vi "ConfigurationFileWrite.vi"() -> ()   [LabVIEW 2016]
uses:
  controls/Enum.ctl
  <vilib>/Utility/config.llb/Write Key (String).vi
  <vilib>/Utility/config.llb/Write Key (Double).vi
  <vilib>/Utility/config.llb/Write Key (Boolean).vi
  <vilib>/Utility/config.llb/Write Key (U32).vi
  <vilib>/Utility/config.llb/Write Key (I32).vi
  <vilib>/Utility/config.llb/NI_LVConfig.lvlib
  <vilib>/Utility/config.llb/Write Key (Path).vi
panel:
  in  "default name":path=path "Configuration File3.ini"
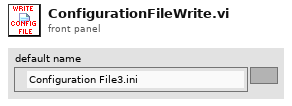
[diagram p1: front panel]
types:
  T1 = typedef "NI_LVConfig.lvlib/Config Data RefNum.ctl" = refnum<k1>
  T2 = typedef "Enum.ctl" = enum16{"Init", "Read", "Write"}
  T3 = enum16{"fractional", "engineering", "exponential"}
  T4 = enum16{"Vert. Deflection", "Horiz. Deflection", "Amplitude", "..."}
  T5 = enum32{"No Selection", "FullScale", "Standard Deviation"}
  T6 = cluster{i32, "Direction":enum16{"Forward", "Backward"}, "Processing":enum16{"None", "Offset", "Line", "Polynom"}, "Color":enum16{"Blue", "Gray", "Gold", "Green", "Red", "Asylum", "Adrian", "Nanoscope", "NanoscopeIII"}}
  T7 = enum32{"Invalid", "Standard", "Closed", "Hidden", "Minimized", "Maximized"}
  T8 = typedef "LVPositionTypeDef.ctl" = cluster{"Left":i32, "Top":i32}
  T9 = cluster{"calibName":string[], "calibParameters":cluster{"Sensitivity":cluster{"Sens X":dbl, "Sens Y":dbl, "Sens Z":dbl}, "Range":cluster{"Range X":dbl, "Range Y":dbl, "Range Z":dbl}, "HV gain":cluster{"HV gain X":dbl, "HV gain Y":dbl, "HV gain Z":dbl}}[], "calibIndex":i32}
  T10 = cluster{"Sensitivity":cluster{"Sens X":dbl, "Sens Y":dbl, "Sens Z":dbl}, "Range":cluster{"Range X":dbl, "Range Y":dbl, "Range Z":dbl}, "HV gain":cluster{"HV gain X":dbl, "HV gain Y":dbl, "HV gain Z":dbl}}[]
  T11 = cluster{"Sensitivity":cluster{"Sens X":dbl, "Sens Y":dbl, "Sens Z":dbl}, "Range":cluster{"Range X":dbl, "Range Y":dbl, "Range Z":dbl}, "HV gain":cluster{"HV gain X":dbl, "HV gain Y":dbl, "HV gain Z":dbl}}
  T12 = cluster{"Sens X":dbl, "Sens Y":dbl, "Sens Z":dbl}
  T13 = cluster{"Range X":dbl, "Range Y":dbl, "Range Z":dbl}
  T14 = cluster{"HV gain X":dbl, "HV gain Y":dbl, "HV gain Z":dbl}
  T15 = cluster{"ActiveController":dbl, "ControllerNames":string[], "ControllerParameters":cluster{"Controller Config":cluster{"Slope":bool, "Controller type":enum16{"Bipolar", "Absolute"}, "Controller name":string, "Control Signal name":string, "Signal":enum16{"Vert. Deflection", "Horiz. Deflection", "Amplitude", "..."}, "Unit":string}, "PID":cluster{"Setpoint":dbl, "P Gain":dbl, "I Gain":dbl}}[]}
  T16 = cluster{"Controller Config":cluster{"Slope":bool, "Controller type":enum16{"Bipolar", "Absolute"}, "Controller name":string, "Control Signal name":string, "Signal":enum16{"Vert. Deflection", "Horiz. Deflection", "Amplitude", "..."}, "Unit":string}, "PID":cluster{"Setpoint":dbl, "P Gain":dbl, "I Gain":dbl}}[]
  T17 = cluster{"Slope":bool, "Controller type":enum16{"Bipolar", "Absolute"}, "Controller name":string, "Control Signal name":string, "Signal":enum16{"Vert. Deflection", "Horiz. Deflection", "Amplitude", "..."}, "Unit":string}
  T18 = cluster{"Setpoint":dbl, "P Gain":dbl, "I Gain":dbl}
  T19 = typedef "ScanWaveform.ctl" = enum16{"Sine Wave", "Triangle Wave", "Rounded Wave"}
  T20 = cluster{"slowWavePts":u16, "fastWavePts":u16, "slowWaveType":T19, "fastWaveType":T19, "slowRoundPts":u16, "fastRoundPts":u16, "singleDirectionScan":bool}
  T21 = cluster{"Width":dbl, "Height":dbl, "X Offset":dbl, "Y Offset":dbl, "Angle":dbl, "Pixels/Line":u16, "Lines":u16, "Time/Line":dbl, "Scan Rate":dbl}
  T22 = enum16{"Blue", "Gray", "Gold", "Green", "Red", "Asylum", "Adrian", "Nanoscope", "NanoscopeIII"}
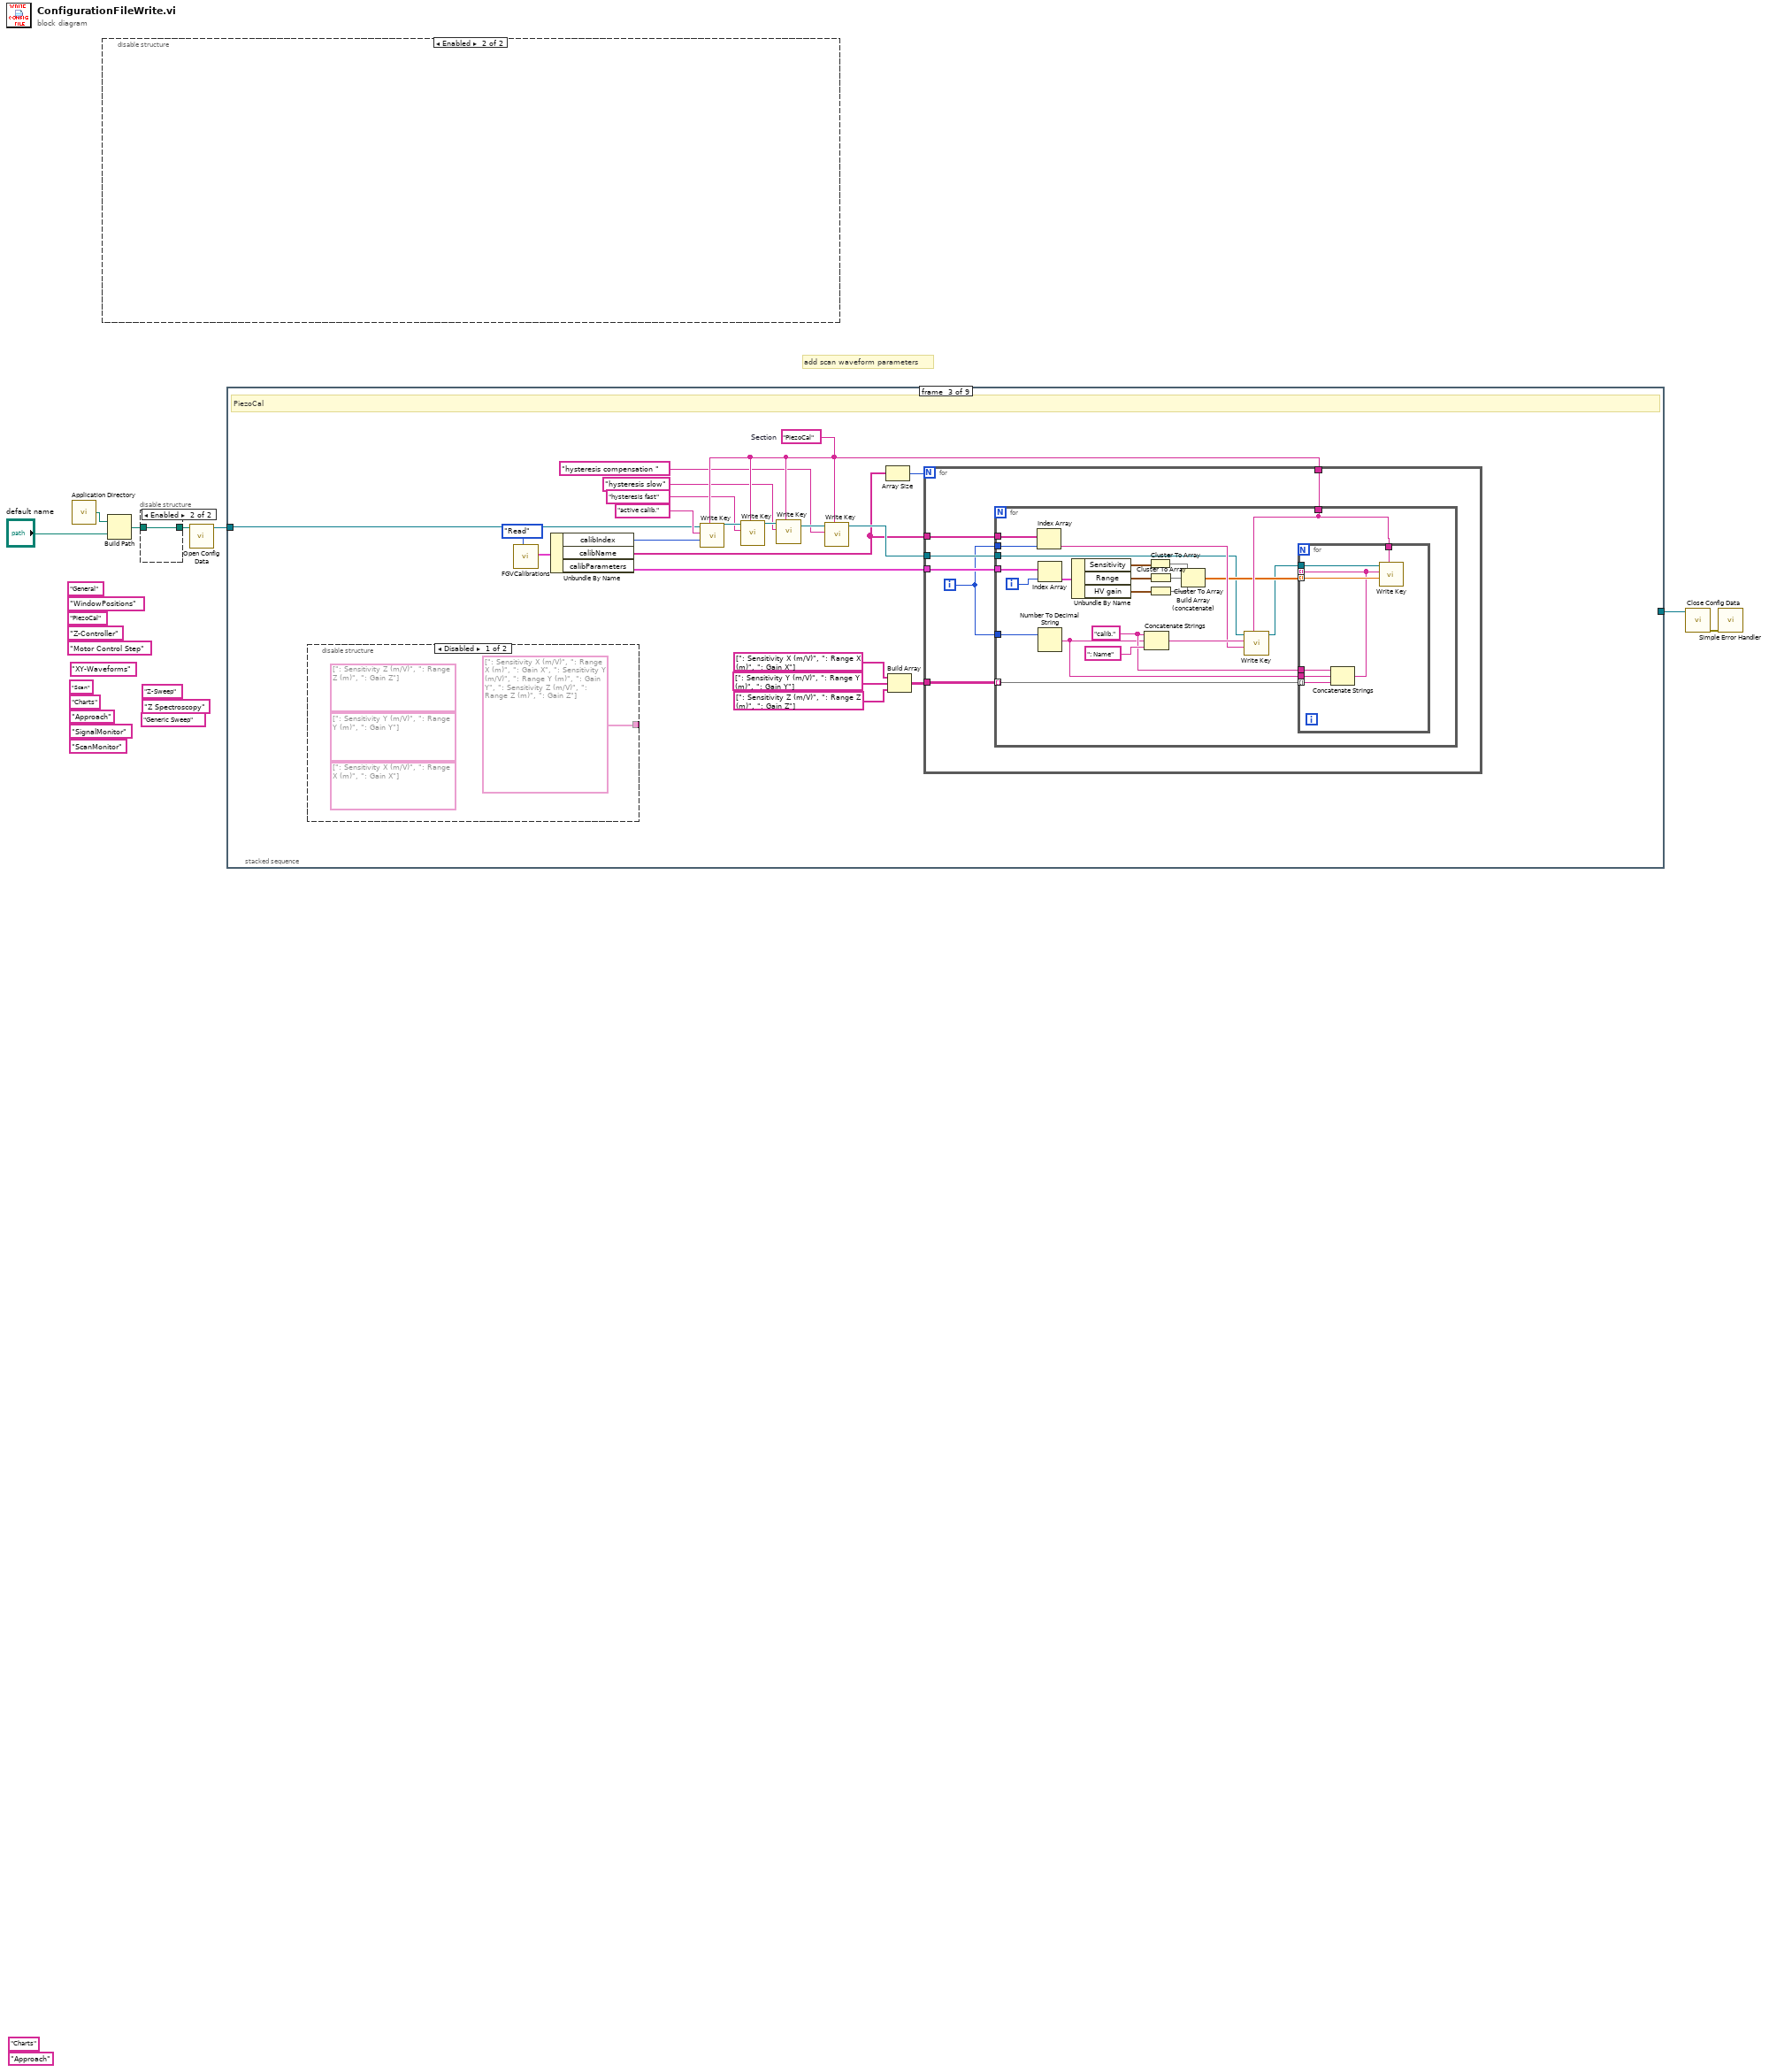
[diagram p0: block diagram]
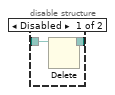
[diagram p2: hidden frame]
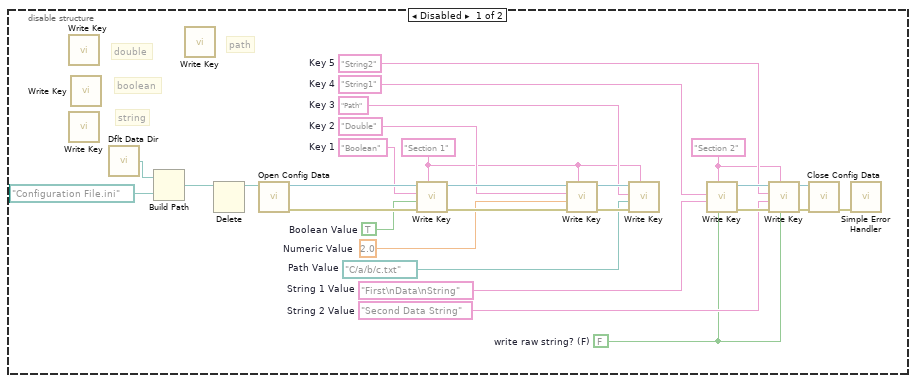
[diagram p3: hidden frame]
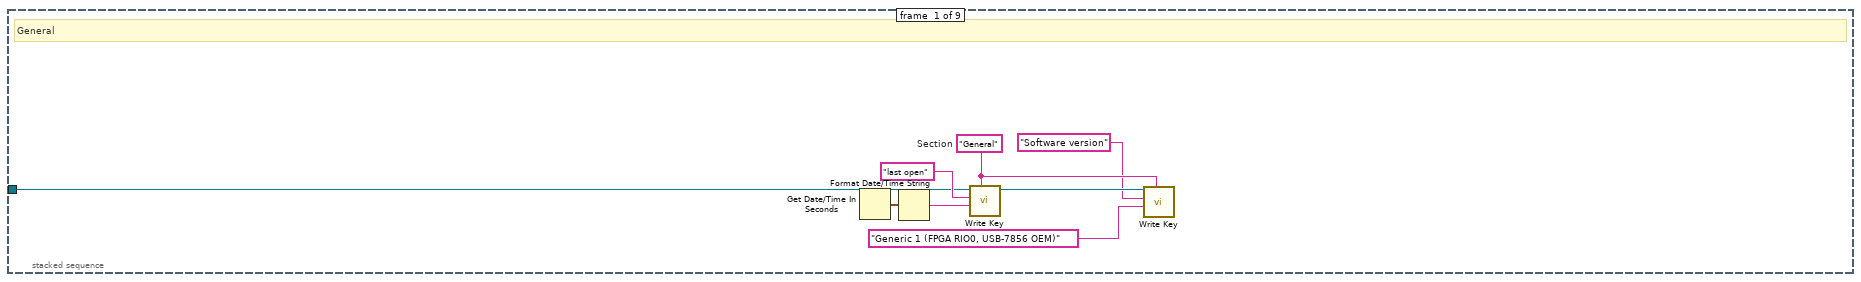
[diagram p4: hidden frame]
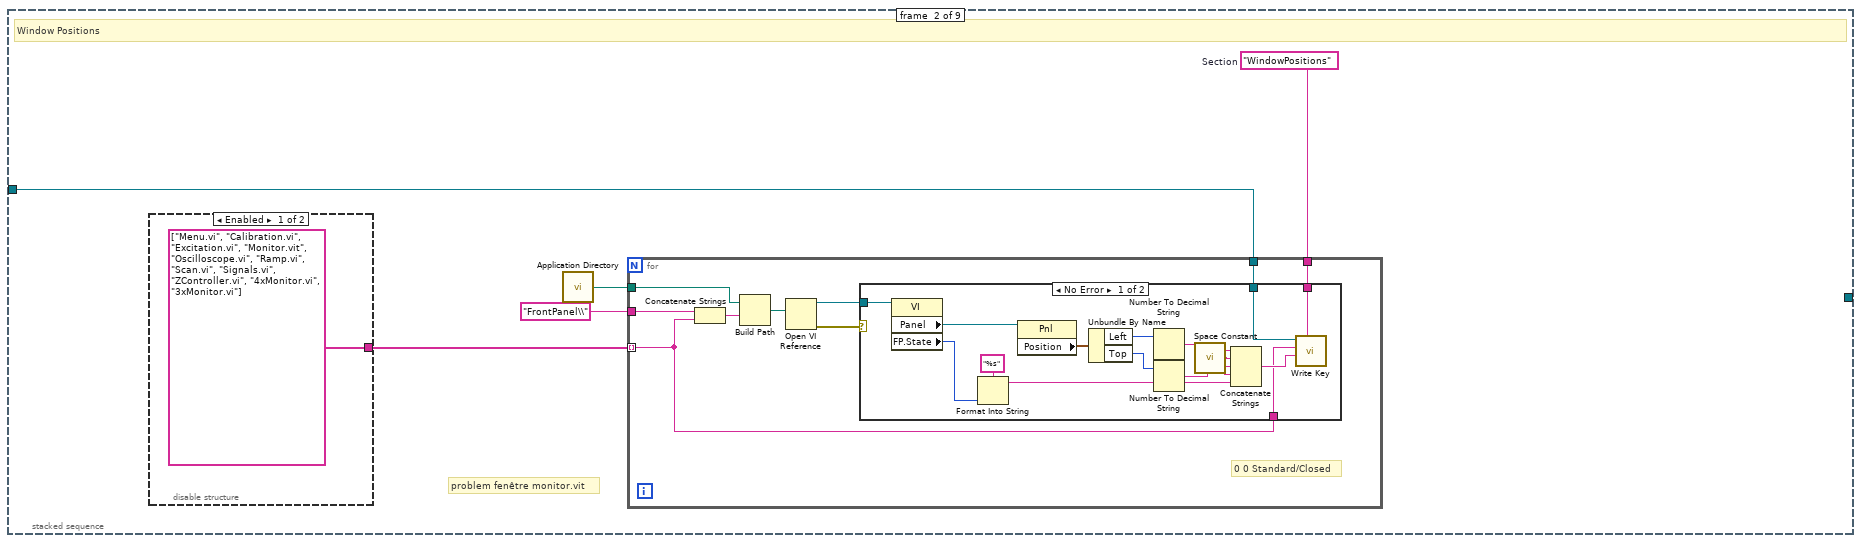
[diagram p5: hidden frame]
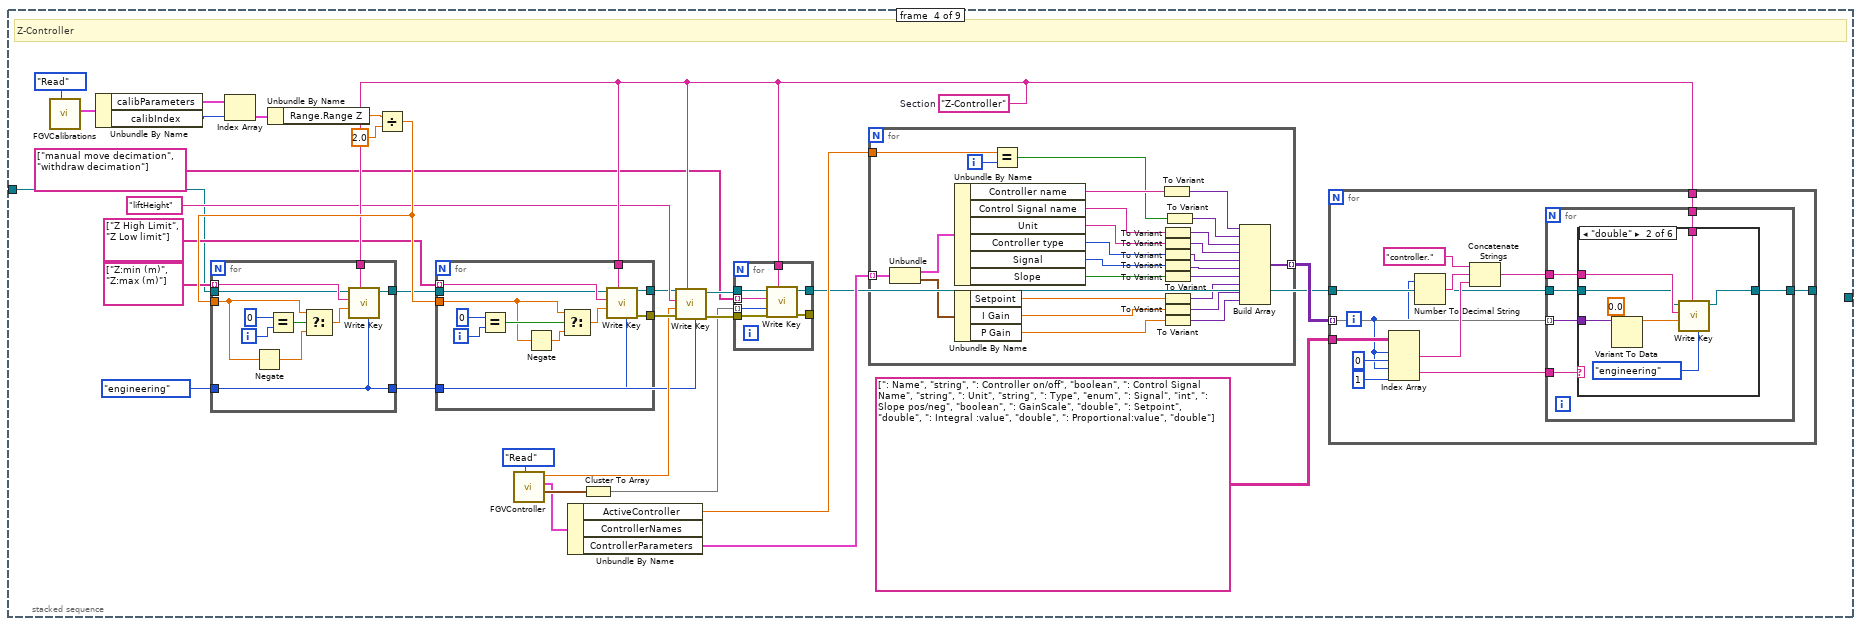
[diagram p9: hidden frame]
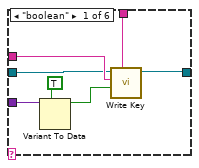
[diagram p10: hidden frame]
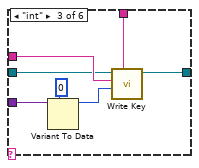
[diagram p11: hidden frame]
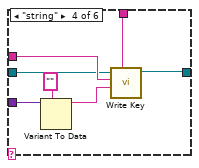
[diagram p12: hidden frame]
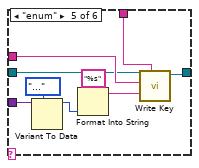
[diagram p13: hidden frame]
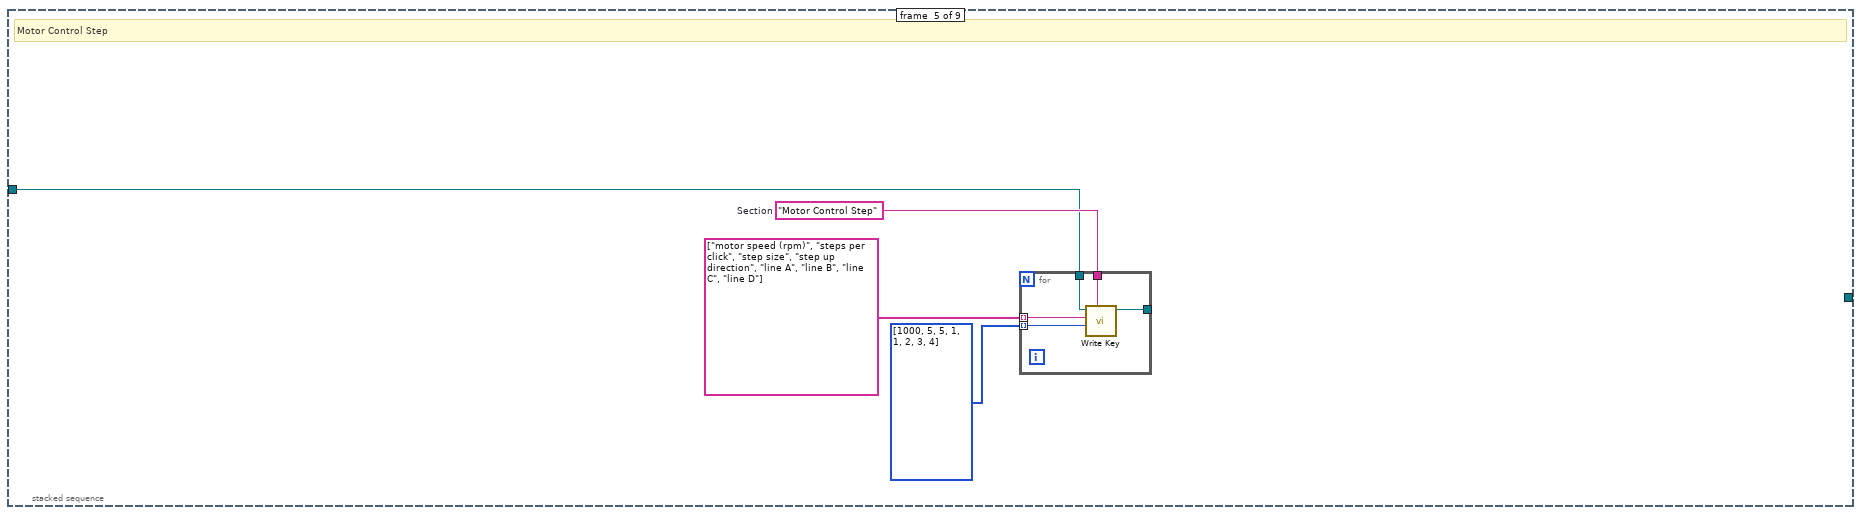
[diagram p15: hidden frame]
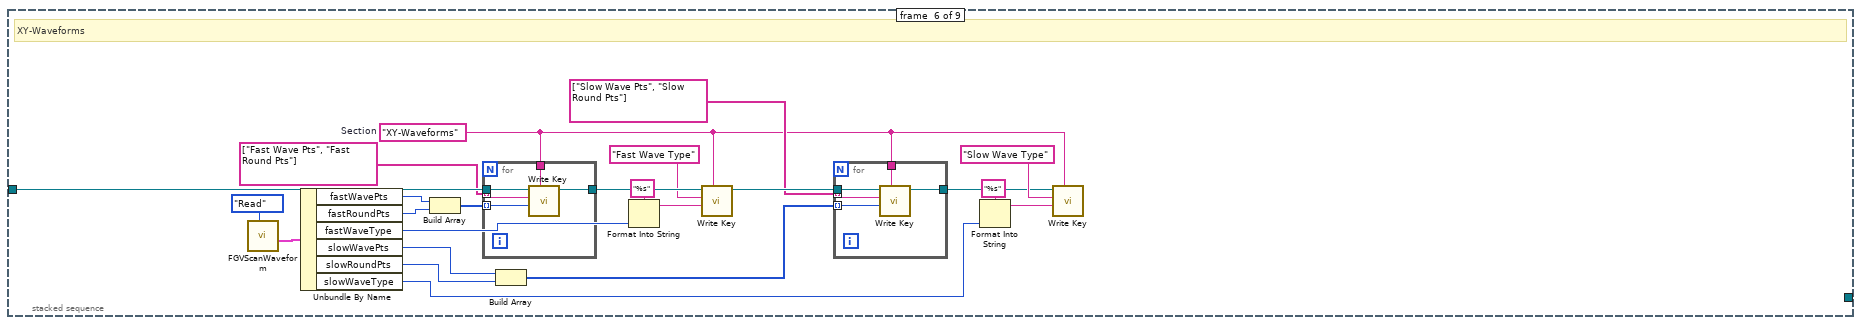
[diagram p16: hidden frame]
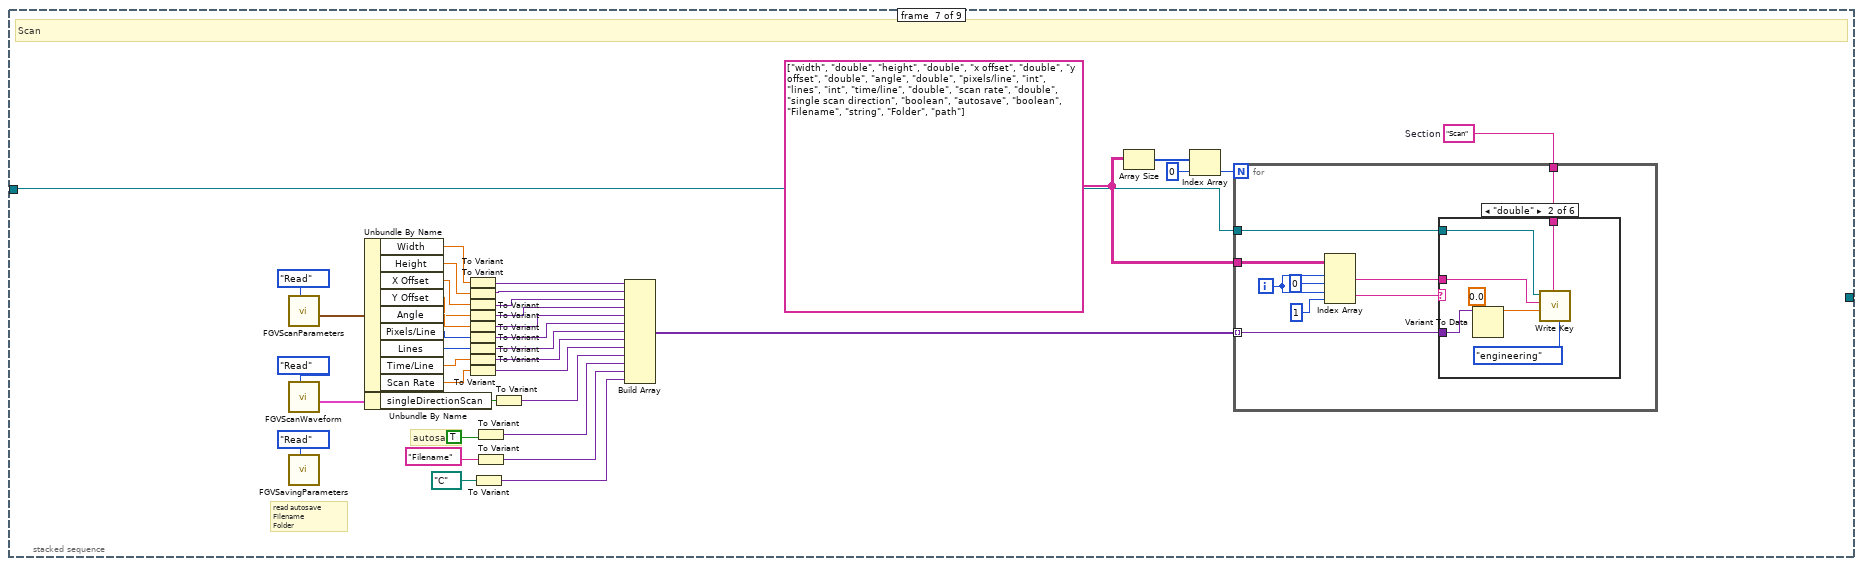
[diagram p17: hidden frame]
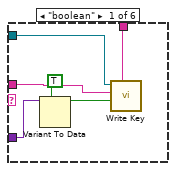
[diagram p18: hidden frame]
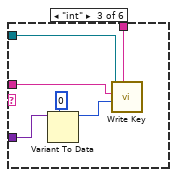
[diagram p19: hidden frame]
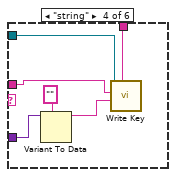
[diagram p20: hidden frame]
diagram:
  (unwired) "XY-Waveforms"
  (unwired) "Approach"
  (unwired) "Charts"
  (unwired) "Generic Sweep"
  (unwired) "ScanMonitor"
  (unwired) "Z Spectroscopy"
  (unwired) "Z-Sweep"
  (unwired) "SignalMonitor"
  (unwired) "Approach"
  (unwired) "Charts"
  (unwired) "Scan"
  (unwired) "Motor Control Step"
  (unwired) "Z-Controller"
  (unwired) "PiezoCal"
  (unwired) "WindowPositions"
  (unwired) "General"
  # "add scan waveform parameters"
  n1 = call <vilib>:"Application Directory.vi"() -> ("Application Directory"=w7:path)
  n2 = disable-structure shown="Enabled" {
    frame Disabled {
      w19 = "Second Data String"  # String 2 Value
      w20 = "First\nData\nString"  # String 1 Value
      w15 = path "C:/a/b/c.txt"  # Path Value
      w14 = 2.0  # Numeric Value
      w13 = TRUE  # Boolean Value
      w8 = FALSE  # write raw string? (F)
      w21 = "String2"  # Key 5
      w22 = "String1"  # Key 4
      w23 = "Path"  # Key 3
      w24 = "Double"  # Key 2
      w25 = "Boolean"  # Key 1
      w16 = "Section 2"
      w17 = "Section 1"
      # "string"
      # "path"
      # "boolean"
      # "double"
      n3 = call-poly <vilib>:"Write Key.vi"() -> ()  [unwired: 8 in, 4 out]
      n4 = call-poly <vilib>:"Write Key.vi"() -> ()  [unwired: 6 in, 6 out]
      n5 = call-poly <vilib>:"Write Key.vi"() -> ()  [unwired: 5 in, 7 out]
      n6 = call <vilib>:"Dflt Data Dir.vi"() -> ("App:Default Data Directory"=w11:path)
      n7 = Build Path(base path=w11, name or relative path=path "Configuration File.ini" ("default name")) -> (appended path=w9:path)
      n8 = call-poly <vilib>:"Write Key.vi"() -> ()  [unwired: 5 in, 7 out]
      n9 = Delete(path (use dialog)=w9) -> (deleted path=w10:path)  [unwired: 4 in, 2 out]
      n10 = call <vilib>:"Open Config Data.vi"("configuration file path"=w10) -> ("error out"=w30:errorcluster, "refnum"=w35:T1)  [unwired: 2 in, 7 out]
      n11 = call-poly <vilib>:"Write Key.vi"("section"=w17, "error in (no error)"=w30, "value"=w13, "key"=w25, "refnum"=w35) -> ("error out"=w29:errorcluster, "refnum out"=w34:T1)  [unwired: 5 out]
      n12 = call-poly <vilib>:"Write Key.vi"("section"=w17, "error in (no error)"=w29, "value"=w14, "key"=w24, "refnum"=w34) -> ("error out"=w28:errorcluster, "refnum out"=w33:T1)  [unwired: 3 in, 2 out]
      n13 = call-poly <vilib>:"Write Key.vi"("section"=w17, "error in (no error)"=w28, "value"=w15, "key"=w23, "refnum"=w33) -> ()  [unwired: 7 out]
      n14 = call-poly <vilib>:"Write Key.vi"("write raw string? (F)"=w8, "section"=w16, "value"=w20, "key"=w22) -> ("error out"=w27:errorcluster, "refnum out"=w32:T1)  [unwired: 2 in, 4 out]
      n15 = call-poly <vilib>:"Write Key.vi"("write raw string? (F)"=w8, "section"=w16, "error in (no error)"=w27, "value"=w19, "key"=w21, "refnum"=w32) -> ("error out"=w26:errorcluster, "refnum out"=w31:T1)  [unwired: 4 out]
      n16 = call <vilib>:"Close Config Data.vi"("error in (no error)"=w26, "refnum"=w31) -> ("error out"=w18:errorcluster)  [unwired: 1 in, 8 out]
      n17 = call <vilib>:"Simple Error Handler.vi"("error in (no error)"=w18) -> ()  [unwired: 1 in, 8 out]
    }
    frame Enabled {
    }
  }
  n18 = Build Path(base path=w7, name or relative path="default name") -> (appended path=w3:path)
  n19 = disable-structure shown="Enabled" {
    disable-tunnel: w3 -> [w37 w38]
    disable-tunnel: [w36 w38] -> w2
    frame Disabled {
      n20 = Delete(path (use dialog)=w37) -> (deleted path=w36:path)  [unwired: 4 in, 2 out]
    }
    frame Enabled {
    }
  }
  n21 = call <vilib>:"Open Config Data.vi"("configuration file path"=w2) -> ("refnum"=w6:T1)  [unwired: 2 in, 8 out]
  n22 = stacked-sequence {
    tunnel: w6 -> [w39 w48 w83 w136 w278 w309 w324 w404 w460]
    tunnel: [_ _ _ _ _ _ _ _ w459] -> w4
    frame #0 {
      w46 = "General"  # Section
      # "General"
      n23 = Get Date/Time In Seconds() -> (seconds since 1Jan1904=w44:timestamp)
      n24 = Format Date/Time String(seconds (now)=w44) -> (date/time string=w45:string)  [unwired: 2 in]
      n25 = call-poly <vilib>:"Write Key.vi"("section"=w46, "value"=w45, "key"="last open", "refnum"=w39) -> ("refnum out"=w43:T1)  [unwired: 2 in, 5 out]
      n26 = call-poly <vilib>:"Write Key.vi"("section"=w46, "value"="Generic 1 (FPGA RIO0, USB-7856 OEM)", "key"="Software version", "refnum"=w43) -> ()  [unwired: 2 in, 6 out]
    }
    frame #1 {
      w51 = "WindowPositions"  # Section
      # "problem fenêtre monitor.vit"
      # "Window Positions"
      n27 = disable-structure shown="Enabled" {
        disable-tunnel: [string[] ["Menu.vi", "Calibration.vi", "Excitation.vi", "Monitor.vit", "Oscilloscope.vi", "Ramp.vi", "Scan.vi", "Signals.vi", "ZController.vi", "4xMonitor.vi", "3xMonitor.vi"] _] -> w47
        frame Enabled {
        }
        frame Disabled {
        }
      }
      n28 = call <vilib>:"Application Directory.vi"() -> ("Application Directory"=w50:path)
      n29 = for {
        tunnel: "FrontPanel\\" ("string") -> [w61]
        tunnel: w50 -> [w58]
        tunnel: w47 -> [w57] mode=indexing
        tunnel: w51 -> [w56]
        tunnel: w48 -> [w54]
        # "0 0 Standard/Closed"
        n30 = Concatenate Strings(w61, w57) -> (w60:string)
        n31 = Build Path(base path=w58, name or relative path=w60) -> (appended path=w59:path)
        n32 = Open VI Reference(vi path=w59) -> (vi reference=w55:refnum<vi>, error out=w53:errorcluster)  [unwired: 5 in]
        n33 = case shown="No Error" w53 {
          tunnel: w57 -> [w69 _]
          tunnel: w56 -> [w68 _]
          tunnel: w55 -> [w67 _]
          tunnel: w54 -> [w62 _]
          frame No Error {
            n34 = property class="VI"(reference=w67) -> ("Panel"=w76:refnum<vi>, "FP.State"=w66:T7)  [unwired: 1 in, 2 out]
            n35 = Format Into String(format string="%s", w66) -> (resulting string=w63:string)  [unwired: 2 in, 1 out]
            n36 = property class="Pnl"(reference=w76) -> ("Position"=w75:T8)  [unwired: 1 in, 2 out]
            n37 = Unbundle By Name(w75) -> ("Left"=w74:i32, "Top"=w73:i32)
            n38 = Number To Decimal String(number=w74) -> (decimal integer string=w72:string)  [unwired: 1 in]
            n39 = Number To Decimal String(number=w73) -> (decimal integer string=w71:string)  [unwired: 1 in]
            n40 = call <vilib>:"Space Constant.vi"() -> ("String"=w64:string)
            n41 = Concatenate Strings(w72, w64, w71, w64, w63) -> (w70:string)
            n42 = call-poly <vilib>:"Write Key.vi"("section"=w68, "value"=w70, "key"=w69, "refnum"=w62) -> ()  [unwired: 2 in, 6 out]
          }
          frame Error {
          }
        }
      }
    }
    frame #2 {
      w94 = "PiezoCal"  # Section
      # "PiezoCal"
      n43 = disable-structure shown="Disabled" {
        disable-tunnel: [string[] [": Sensitivity X (m/V)", ": Range X (m)", ": Gain X", ": Sensitivity Y (m/V)", ": Range Y (m)", ": Gain Y", ": Sensitivity Z (m/V)", ": Range Z (m)", ": Gain Z"] ("Array") _] -> _
        frame Disabled {
          (unwired) string[] [": Sensitivity X (m/V)", ": Range X (m)", ": Gain X"] ("Array")
          (unwired) string[] [": Sensitivity Z (m/V)", ": Range Z (m)", ": Gain Z"] ("Array")
          (unwired) string[] [": Sensitivity Y (m/V)", ": Range Y (m)", ": Gain Y"] ("Array")
        }
        frame Enabled {
        }
      }
      n44 = call "FGVCalibrations.vi"("Enum"=Enum."Read") -> ("calibOut"=w86:T9)  [unwired: 9 in, 1 out]
      n45 = Unbundle By Name(w86) -> ("calibIndex"=w96:i32, "calibName"=w81:string[], "calibParameters"=w95:T10)
      n46 = call-poly <vilib>:"Write Key.vi"("section"=w94, "value"=w96, "key"="active calib.", "refnum"=w83) -> ("refnum out"=w93:T1)  [unwired: 4 in, 3 out]
      n47 = call-poly <vilib>:"Write Key.vi"("section"=w94, "key"="hysteresis fast", "refnum"=w93) -> ("refnum out"=w92:T1)  [unwired: 2 in, 6 out]
      n48 = call-poly <vilib>:"Write Key.vi"("section"=w94, "key"="hysteresis slow", "refnum"=w92) -> ("refnum out"=w91:T1)  [unwired: 2 in, 6 out]
      n49 = call-poly <vilib>:"Write Key.vi"("section"=w94, "key"="hysteresis compensation ", "refnum"=w91) -> ("refnum out"=w84:T1)  [unwired: 2 in, 6 out]
      n50 = Array Size(array=w81) -> (size(s)=w82:i32)
      n51 = Build Array(string[] [": Sensitivity X (m/V)", ": Range X (m)", ": Gain X"] ("Array"), string[] [": Sensitivity Y (m/V)", ": Range Y (m)", ": Gain Y"] ("Array"), string[] [": Sensitivity Z (m/V)", ": Range Z (m)", ": Gain Z"] ("Array")) -> (w80:string[][])
      n52 = for {
        N: w82 -> [_]
        tunnel: w95 -> [w103]
        tunnel: w80 -> [w102]
        tunnel: w94 -> [w101]
        tunnel: w81 -> [w99]
        tunnel: w84 -> [w100]
        i -> [w98]
        n53 = for {
          tunnel: w99 -> [w125]
          tunnel: w103 -> [w121]
          tunnel: w101 -> [w119]
          tunnel: w102 -> [w104] mode=indexing
          tunnel: w100 -> [w111]
          tunnel: w98 -> [w109]
          tunnel: w98 -> [w108]
          i -> [w107]
          w106 = "calib."
          n54 = Index Array(array=w125, index=w108) -> (element=w122:string)
          n55 = Index Array(array=w121, index=w107) -> (element=w120:T11)
          n56 = Number To Decimal String(number=w109) -> (decimal integer string=w105:string)  [unwired: 1 in]
          n57 = Unbundle By Name(w120) -> ("Sensitivity"=w118:T12, "Range"=w116:T13, "HV gain"=w117:T14)
          n58 = Concatenate Strings(w106, w105, ": Name") -> (w123:string)
          n59 = Cluster To Array(cluster=w118) -> (array=w115:dbl[])
          n60 = Cluster To Array(cluster=w116) -> (array=w114:dbl[])
          n61 = Cluster To Array(cluster=w117) -> (array=w113:dbl[])
          n62 = Build Array (concatenate)(w115, w114, w113) -> (w112:dbl[])
          n63 = call-poly <vilib>:"Write Key.vi"("section"=w119, "value"=w122, "key"=w123, "refnum"=w111) -> ("refnum out"=w110:T1)  [unwired: 2 in, 5 out]
          n64 = for {
            tunnel: [w126] -> _ mode=indexing
            tunnel: w119 -> [w132]
            tunnel: w112 -> [w131] mode=indexing
            tunnel: w110 -> [w130]
            tunnel: w106 -> [w129]
            tunnel: w105 -> [w128]
            tunnel: w104 -> [w127] mode=indexing
            n65 = Concatenate Strings(w129, w128, w127) -> (w126:string)
            n66 = call-poly <vilib>:"Write Key.vi"("section"=w132, "value"=w131, "key"=w126, "refnum"=w130) -> ()  [unwired: 4 in, 4 out]
          }
        }
      }
    }
    frame #3 {
      w153 = "Z-Controller"  # Section
      # "Z-Controller"
      n67 = call "FGVCalibrations.vi"("Enum"=Enum."Read") -> ("calibOut"=w156:T9)  [unwired: 9 in, 1 out]
      n68 = Unbundle By Name(w156) -> ("calibParameters"=w157:T10, "calibIndex"=w158:i32)
      n69 = Index Array(array=w157, index=w158) -> (element=w138:T11)
      n70 = Unbundle By Name(w138) -> ("Range.Range Z"=w137:dbl)
      n71 = Divide(x=w137, y=2.0) -> (x/y=w162:dbl)
      n72 = for {
        tunnel: string[] ["Z:min (m)", "Z:max (m)"] -> [w273] mode=indexing
        tunnel: w162 -> [w271]
        tunnel: w153 -> [w270]
        tunnel: [w269] -> w142
        tunnel: w136 -> [w268]
        tunnel: T3."engineering" ("format (fractional)") -> [w267]
        tunnel: [w267] -> w133
        i -> [w275]
        n73 = Negate(x=w271) -> (-x=w272:dbl)
        n74 = Equal?(x=0, y=w275) -> (x = y?=w276:bool)
        n75 = Select(t=w271, s=w276, f=w272) -> (s? t:f=w277:dbl)
        n76 = call-poly <vilib>:"Write Key.vi"("format (fractional)"=w267, "section"=w270, "value"=w277, "key"=w273, "refnum"=w268) -> ("refnum out"=w269:T1)  [unwired: 3 in, 3 out]
      }
      n77 = for {
        tunnel: string[] ["Z High Limit", "Z Low limit"] -> [w262] mode=indexing
        tunnel: w162 -> [w260]
        tunnel: w153 -> [w259]
        tunnel: [w258] -> w150
        tunnel: w142 -> [w257]
        tunnel: [w256] -> w163
        tunnel: w133 -> [w255]
        i -> [w264]
        n78 = Equal?(x=0, y=w264) -> (x = y?=w265:bool)
        n79 = Negate(x=w260) -> (-x=w261:dbl)
        n80 = Select(t=w260, s=w265, f=w261) -> (s? t:f=w266:dbl)
        n81 = call-poly <vilib>:"Write Key.vi"("format (fractional)"=w255, "section"=w259, "value"=w266, "key"=w262, "refnum"=w257) -> ("error out"=w256:errorcluster, "refnum out"=w258:T1)  [unwired: 3 in, 2 out]
      }
      n82 = call "FGVController.vi"("Enum"=Enum."Read") -> ("ManualMotionDecOut"=w146:cluster{"WithdrawDec":u16, "ManualMoveDec":u16}, "calibOut"=w144:T15, "liftHeightOut"=w152:dbl)  [unwired: 6 in, 2 out]
      n83 = Unbundle By Name(w144) -> ("ActiveController"=w159:dbl, "ControllerParameters"=w160:T16)  [unwired: 1 out]
      n84 = Cluster To Array(cluster=w146) -> (array=w147:u16[])
      n85 = call-poly <vilib>:"Write Key.vi"("format (fractional)"=w133, "section"=w153, "error in (no error)"=w163, "value"=w152, "key"="liftHeight", "refnum"=w150) -> ("error out"=w148:errorcluster, "refnum out"=w149:T1)  [unwired: 2 in, 2 out]
      n86 = for {
        tunnel: w153 -> [w196]
        tunnel: w149 -> [w195]
        tunnel: w148 -> [w194]
        tunnel: string[] ["manual move decimation", "withdraw decimation"] -> [w193] mode=indexing
        tunnel: w147 -> [w192] mode=indexing
        tunnel: [w191] -> _
        tunnel: [w190] -> w135
        n87 = call-poly <vilib>:"Write Key.vi"("section"=w196, "error in (no error)"=w194, "value"=w192, "key"=w193, "refnum"=w195) -> ("error out"=w191:errorcluster, "refnum out"=w190:T1)  [unwired: 3 in, 2 out]
      }
      n88 = for {
        tunnel: w160 -> [w189] mode=indexing
        tunnel: w159 -> [w167]
        tunnel: [w164] -> w154 mode=indexing
        i -> [w168]
        n89 = Unbundle(w189) -> ("Controller Config"=w188:T17, "PID"=w187:T18)
        n90 = Unbundle By Name(w188) -> ("Controller name"=w186:string, "Control Signal name"=w185:string, "Unit"=w184:string, "Controller type"=w183:enum16{"Bipolar", "Absolute"}, "Signal"=w182:T4, "Slope"=w181:bool)
        n91 = Unbundle By Name(w187) -> ("Setpoint"=w180:dbl, "I Gain"=w179:dbl, "P Gain"=w178:dbl)
        n92 = Equal?(x=w167, y=w168) -> (x = y?=w166:bool)
        n93 = To Variant(anything=w186) -> (Variant=w177:variant)
        n94 = To Variant(anything=w185) -> (Variant=w176:variant)
        n95 = To Variant(anything=w184) -> (Variant=w175:variant)
        n96 = To Variant(anything=w183) -> (Variant=w174:variant)
        n97 = To Variant(anything=w182) -> (Variant=w173:variant)
        n98 = To Variant(anything=w181) -> (Variant=w172:variant)
        n99 = To Variant(anything=w180) -> (Variant=w171:variant)
        n100 = To Variant(anything=w179) -> (Variant=w170:variant)
        n101 = To Variant(anything=w178) -> (Variant=w169:variant)
        n102 = To Variant(anything=w166) -> (Variant=w165:variant)
        n103 = Build Array(w177, w165, w176, w175, w174, w173, w172, w171, w170, w169) -> (w164:variant[])
      }
      n104 = for {
        tunnel: string[][] [[": Name", "string"], [": Controller on/off", "boolean"], [": Control Signal Name", "string"], [": Unit", "string"], [": Type", "enum"], [": Signal", "int"], [": Slope pos/neg", "boolean"], [": GainScale", "double"], [": Setpoint", "double"], [": Integral :value", "double"], [": Proportional:value", "double"]] ("appended array") -> [w205]
        tunnel: w154 -> [w200] mode=indexing
        tunnel: w153 -> [w202]
        tunnel: w135 -> [w198]
        tunnel: [w199] -> _
        i -> [w197]
        n105 = Index Array(array=w205, index (row) #1=w197, index (col) #1=0 ("disabled index (col)"), index (row) #2=w197, index (col) #2=1 ("disabled index (col)")) -> (element #1=w207:string, element #2=w203:string)
        n106 = Number To Decimal String(number=w197) -> (decimal integer string=w208:string)  [unwired: 1 in]
        n107 = Concatenate Strings("controller.", w208, w207) -> (w201:string)
        n108 = for {
          tunnel: w203 -> [w215]
          tunnel: w202 -> [w214]
          tunnel: w201 -> [w213]
          tunnel: w200 -> [w212] mode=indexing
          tunnel: w198 -> [w210]
          tunnel: [w211] -> w199
          n109 = case shown="\"double\"" w215 {
            tunnel: w214 -> [w219 w226 w233 w244 w253 _]
            tunnel: w213 -> [w218 w227 w234 w243 w252 _]
            tunnel: w212 -> [w222 w229 w236 w240 w251 _]
            tunnel: [w216 w224 w232 w239 w245 w254] -> w211
            tunnel: w210 -> [w217 w225 w231 w238 w246 w254]
            frame "boolean" {
              n110 = Variant To Data(type=TRUE, Variant=w222) -> (data=w220:bool)  [unwired: 1 in, 1 out]
              n111 = call-poly <vilib>:"Write Key.vi"("section"=w219, "value"=w220, "key"=w218, "refnum"=w217) -> ("refnum out"=w216:T1)  [unwired: 1 in, 6 out]
            }
            frame "double" {
              n112 = Variant To Data(type=0.0 ("Signal"), Variant=w229) -> (data=w228:dbl)  [unwired: 1 in, 1 out]
              n113 = call-poly <vilib>:"Write Key.vi"("format (fractional)"=T3."engineering", "section"=w226, "value"=w228, "key"=w227, "refnum"=w225) -> ("refnum out"=w224:T1)  [unwired: 3 in, 3 out]
            }
            frame "int" {
              n114 = Variant To Data(type=u16 0 ("Signal"), Variant=w236) -> (data=w235:u16)  [unwired: 1 in, 1 out]
              n115 = call-poly <vilib>:"Write Key.vi"("section"=w233, "value"=w235, "key"=w234, "refnum"=w231) -> ("refnum out"=w232:T1)  [unwired: 1 in, 6 out]
            }
            frame "string" {
              n116 = Variant To Data(type="", Variant=w240) -> (data=w241:string)  [unwired: 1 in, 1 out]
              n117 = call-poly <vilib>:"Write Key.vi"("section"=w244, "value"=w241, "key"=w243, "refnum"=w238) -> ("refnum out"=w239:T1)  [unwired: 2 in, 5 out]
            }
            frame "enum" {
              n118 = Variant To Data(type=T4."..." ("Signal"), Variant=w251) -> (data=w249:T4)  [unwired: 1 in, 1 out]
              n119 = Format Into String(format string="%s", w249) -> (resulting string=w247:string)  [unwired: 2 in, 1 out]
              n120 = call-poly <vilib>:"Write Key.vi"("section"=w253, "value"=w247, "key"=w252, "refnum"=w246) -> ("refnum out"=w245:T1)  [unwired: 2 in, 5 out]
            }
            frame Default {
            }
          }
        }
      }
    }
    frame #4 {
      w281 = "Motor Control Step"  # Section
      # "Motor Control Step"
      n121 = for {
        tunnel: string[] ["motor speed (rpm)", "steps per click", "step size", "step up direction", "line A", "line B", "line C", "line D"] -> [w286] mode=indexing
        tunnel: i32[] [1000, 5, 5, 1, 1, 2, 3, 4] ("number") -> [w285] mode=indexing
        tunnel: w281 -> [w284]
        tunnel: [w283] -> _
        tunnel: w278 -> [w282]
        n122 = call-poly <vilib>:"Write Key.vi"("section"=w284, "value"=w285, "key"=w286, "refnum"=w282) -> ("refnum out"=w283:T1)  [unwired: 1 in, 6 out]
      }
    }
    frame #5 {
      w290 = "XY-Waveforms"  # Section
      # "XY-Waveforms"
      n123 = call "FGVScanWaveform.vi"("Enum"=Enum."Read") -> ("scanWaveFormCtl Out"=w307:T20)  [unwired: 9 in, 1 out]
      n124 = Unbundle By Name(w307) -> ("fastWavePts"=w306:u16, "fastRoundPts"=w305:u16, "fastWaveType"=w303:T19, "slowWavePts"=w289:u16, "slowRoundPts"=w288:u16, "slowWaveType"=w287:T19)
      n125 = Build Array(w306, w305) -> (w304:u16[])
      n126 = for {
        tunnel: w304 -> [w319] mode=indexing
        tunnel: string[] ["Fast Wave Pts", "Fast Round Pts"] -> [w318] mode=indexing
        tunnel: w290 -> [w317]
        tunnel: [w316] -> w301
        tunnel: w309 -> [w315]
        n127 = call-poly <vilib>:"Write Key.vi"("section"=w317, "value"=w319, "key"=w318, "refnum"=w315) -> ("refnum out"=w316:T1)  [unwired: 1 in, 6 out]
      }
      n128 = Build Array(w289, w288) -> (w292:u16[])
      n129 = Format Into String(format string="%s", w303) -> (resulting string=w300:string)  [unwired: 2 in, 1 out]
      n130 = call-poly <vilib>:"Write Key.vi"("section"=w290, "value"=w300, "key"="Fast Wave Type", "refnum"=w301) -> ("refnum out"=w293:T1)  [unwired: 2 in, 5 out]
      n131 = for {
        tunnel: w292 -> [w314] mode=indexing
        tunnel: string[] ["Slow Wave Pts", "Slow Round Pts"] -> [w313] mode=indexing
        tunnel: w290 -> [w312]
        tunnel: [w311] -> w295
        tunnel: w293 -> [w310]
        n132 = call-poly <vilib>:"Write Key.vi"("section"=w312, "value"=w314, "key"=w313, "refnum"=w310) -> ("refnum out"=w311:T1)  [unwired: 1 in, 6 out]
      }
      n133 = Format Into String(format string="%s", w287) -> (resulting string=w296:string)  [unwired: 2 in, 1 out]
      n134 = call-poly <vilib>:"Write Key.vi"("section"=w290, "value"=w296, "key"="Slow Wave Type", "refnum"=w295) -> ()  [unwired: 2 in, 6 out]
    }
    frame #6 {
      w323 = string[][] [["width", "double"], ["height", "double"], ["x offset", "double"], ["y offset", "double"], ["angle", "double"], ["pixels/line", "int"], ["lines", "int"], ["time/line", "double"], ["scan rate", "double"], ["single scan direction", "boolean"], ["autosave", "boolean"], ["Filename", "string"], ["Folder", "path"]] ("transposed array")
      w347 = "Scan"  # Section
      # "read autosave\nFilename\nFolder"
      # "autosave"
      # "Scan"
      n135 = call "FGVScanParameters.vi"("Enum"=Enum."Read") -> ("Scan Parameters Out"=w327:T21)  [unwired: 9 in, 1 out]
      n136 = call "FGVScanWaveform.vi"("Enum"=Enum."Read") -> ("scanWaveFormCtl Out"=w349:T20)  [unwired: 9 in, 1 out]
      n137 = call "FGVSavingParameters.vi"("Enum"=Enum."Read") -> ()  [unwired: 7 in, 4 out]
      n138 = Unbundle By Name(w327) -> ("Width"=w337:dbl, "Height"=w338:dbl, "X Offset"=w339:dbl, "Y Offset"=w340:dbl, "Angle"=w341:dbl, "Pixels/Line"=w342:u16, "Lines"=w343:u16, "Time/Line"=w344:dbl, "Scan Rate"=w345:dbl)
      n139 = Unbundle By Name(w349) -> ("singleDirectionScan"=w350:bool)
      n140 = To Variant(anything=w337) -> (Variant=w328:variant)
      n141 = To Variant(anything=w338) -> (Variant=w336:variant)
      n142 = To Variant(anything=w339) -> (Variant=w329:variant)
      n143 = To Variant(anything=w340) -> (Variant=w330:variant)
      n144 = To Variant(anything=w341) -> (Variant=w331:variant)
      n145 = To Variant(anything=w342) -> (Variant=w332:variant)
      n146 = To Variant(anything=w343) -> (Variant=w333:variant)
      n147 = To Variant(anything=w344) -> (Variant=w334:variant)
      n148 = To Variant(anything=w345) -> (Variant=w335:variant)
      n149 = To Variant(anything=path "C:/") -> (Variant=w357:variant)
      n150 = To Variant(anything=TRUE) -> (Variant=w355:variant)
      n151 = To Variant(anything="Filename") -> (Variant=w356:variant)
      n152 = To Variant(anything=w350) -> (Variant=w351:variant)
      n153 = Build Array(w328, w336, w329, w330, w331, w332, w333, w334, w335, w351, w355, w356, w357) -> (w346:variant[])
      n154 = Array Size(array=w323) -> (size(s)=w322:i32[])
      n155 = Index Array(array=w322, index=0) -> (element=w321:i32)
      n156 = for {
        N: w321 -> [_]
        tunnel: w323 -> [w364]
        tunnel: w346 -> [w366] mode=indexing
        tunnel: w347 -> [w365]
        tunnel: w324 -> [w358]
        i -> [w361]
        n157 = Index Array(array=w364, index (row) #1=w361, index (col) #1=0 ("disabled index (col)"), index (row) #2=w361, index (col) #2=1 ("disabled index (col)")) -> (element #1=w362:string, element #2=w359:string)
        n158 = case shown="\"double\"" w359 {
          tunnel: w366 -> [w370 w377 w383 w389 w395 _]
          tunnel: w365 -> [w369 w375 w382 w387 w394 _]
          tunnel: w362 -> [w368 w374 w381 w388 w393 _]
          tunnel: w358 -> [w367 w376 w380 w386 w392 _]
          frame "boolean" {
            n159 = Variant To Data(type=TRUE, Variant=w370) -> (data=w371:bool)  [unwired: 1 in, 1 out]
            n160 = call-poly <vilib>:"Write Key.vi"("section"=w369, "value"=w371, "key"=w368, "refnum"=w367) -> ()  [unwired: 1 in, 7 out]
          }
          frame "double" {
            n161 = Variant To Data(type=0.0 ("Signal"), Variant=w377) -> (data=w378:dbl)  [unwired: 1 in, 1 out]
            n162 = call-poly <vilib>:"Write Key.vi"("format (fractional)"=T3."engineering", "section"=w375, "value"=w378, "key"=w374, "refnum"=w376) -> ()  [unwired: 3 in, 4 out]
          }
          frame "int" {
            n163 = Variant To Data(type=u32 0 ("Signal"), Variant=w383) -> (data=w384:u32)  [unwired: 1 in, 1 out]
            n164 = call-poly <vilib>:"Write Key.vi"("section"=w382, "value"=w384, "key"=w381, "refnum"=w380) -> ()  [unwired: 1 in, 7 out]
          }
          frame "string" {
            n165 = Variant To Data(type="", Variant=w389) -> (data=w390:string)  [unwired: 1 in, 1 out]
            n166 = call-poly <vilib>:"Write Key.vi"("section"=w387, "value"=w390, "key"=w388, "refnum"=w386) -> ()  [unwired: 2 in, 6 out]
          }
          frame "enum" {
            n167 = Variant To Data(type=T4."..." ("Signal"), Variant=w395) -> (data=w398:T4)  [unwired: 1 in, 1 out]
            n168 = Format Into String(format string="%s", w398) -> (resulting string=w396:string)  [unwired: 2 in, 1 out]
            n169 = call-poly <vilib>:"Write Key.vi"("section"=w394, "value"=w396, "key"=w393, "refnum"=w392) -> ()  [unwired: 2 in, 6 out]
          }
          frame Default {
          }
        }
      }
    }
    frame #7 {
      w403 = string[][] [["Channel", "int"], ["Direction", "enum"], ["Processing", "enum"], ["Color", "enum"], ["noSelection/fullScale/standardDev", "enum"]] ("transposed array")
      w405 = "ScanMonitor"  # Section
      # "bug enum"
      # "Direction: int--> enum"
      # "Scan Monitor"
      n170 = Unbundle(T6 {0, "Direction"=enum."Forward", "Processing"=enum."None", "Color"=enum."Blue"} ("Controls")) -> (w411:i32, "Direction"=w412:enum16{"Forward", "Backward"}, "Processing"=w413:enum16{"None", "Offset", "Line", "Polynom"}, "Color"=w414:T22)
      n171 = To Variant(anything=T5."FullScale" ("ZScale")) -> (Variant=w416:variant)
      n172 = To Variant(anything=w411) -> (Variant=w406:variant)
      n173 = To Variant(anything=w412) -> (Variant=w409:variant)
      n174 = To Variant(anything=w413) -> (Variant=w408:variant)
      n175 = To Variant(anything=w414) -> (Variant=w407:variant)
      n176 = Array Size(array=w403) -> (size(s)=w401:i32[])
      n177 = Build Array(w406, w409, w408, w407, w416) -> (w415:variant[])
      n178 = Index Array(array=w401, index=0) -> (element=w402:i32)
      n179 = for {
        N: w402 -> [_]
        tunnel: w403 -> [w425]
        tunnel: w405 -> [w426]
        tunnel: w415 -> [w419] mode=indexing
        tunnel: w404 -> [w418]
        i -> [w422]
        (unwired) enum16{"Forward", "Backward"}."Forward" ("Direction")
        n180 = Index Array(array=w425, index (row) #1=w422, index (col) #1=0 ("disabled index (col)"), index (row) #2=w422, index (col) #2=1 ("disabled index (col)")) -> (element #1=w423:string, element #2=w420:string)
        n181 = case shown="\"enum\"" w420 {
          tunnel: w426 -> [w429 w434 w442 w447 w453 _]
          tunnel: w423 -> [w428 w435 w441 w446 w454 _]
          tunnel: w419 -> [w430 w436 w440 w448 w455 _]
          tunnel: w418 -> [w427 w433 w439 w445 w452 _]
          frame "boolean" {
            n182 = Variant To Data(type=TRUE, Variant=w430) -> (data=w431:bool)  [unwired: 1 in, 1 out]
            n183 = call-poly <vilib>:"Write Key.vi"("section"=w429, "value"=w431, "key"=w428, "refnum"=w427) -> ()  [unwired: 1 in, 7 out]
          }
          frame "double" {
            n184 = Variant To Data(type=0.0 ("Signal"), Variant=w436) -> (data=w437:dbl)  [unwired: 1 in, 1 out]
            n185 = call-poly <vilib>:"Write Key.vi"("section"=w434, "value"=w437, "key"=w435, "refnum"=w433) -> ()  [unwired: 4 in, 4 out]
          }
          frame "int" {
            n186 = Variant To Data(type=u32 0 ("Signal"), Variant=w440) -> (data=w443:u32)  [unwired: 1 in, 1 out]
            n187 = call-poly <vilib>:"Write Key.vi"("section"=w442, "value"=w443, "key"=w441, "refnum"=w439) -> ()  [unwired: 1 in, 7 out]
          }
          frame "string" {
            n188 = Variant To Data(type="", Variant=w448) -> (data=w449:string)  [unwired: 1 in, 1 out]
            n189 = call-poly <vilib>:"Write Key.vi"("section"=w447, "value"=w449, "key"=w446, "refnum"=w445) -> ()  [unwired: 2 in, 6 out]
          }
          frame "enum" {
            n190 = Variant To Data(type=enum16{""}."", Variant=w455) -> (data=w458:enum16{""})  [unwired: 1 in, 1 out]
            n191 = Format Into String(format string="%s", w458) -> (resulting string=w456:string)  [unwired: 2 in, 1 out]
            n192 = call-poly <vilib>:"Write Key.vi"("section"=w453, "value"=w456, "key"=w454, "refnum"=w452) -> ()  [unwired: 2 in, 6 out]
          }
          frame Default {
          }
        }
      }
    }
    frame #8 {
      w468 = i32[] [0, 0, 0, 0, 0, 0, 0, 0]  # Offset
      w467 = i32[] [-1, 1, 1, 1, 1, 1, 1, 1]  # Cal
      w463 = string[] ["m", "V", "V", "V", "V", "V", "V", ""]  # Unit
      w461 = string[] ["Height", "Vert. Deflection", "Horiz. Deflection", "Channel 4", "Channel 5", "Channel 6", "AuxIn", "Obelix"]  # Name
      w469 = "SignalMonitor"  # Section
      # "replace by fgv Signals"
      # "Signal Monitor"
      n193 = for {
        tunnel: w461 -> [w489] mode=indexing
        tunnel: "channel " -> [w488]
        tunnel: w463 -> [w479] mode=indexing
        tunnel: "unit " -> [w486]
        tunnel: "cal " -> [w485]
        tunnel: "offset " -> [w484]
        tunnel: w467 -> [w478] mode=indexing
        tunnel: w468 -> [w477] mode=indexing
        tunnel: w469 -> [w476]
        tunnel: w460 -> [w475]
        tunnel: [w471] -> w459
        i -> [w470]
        n194 = Number To Decimal String(number=w470) -> (decimal integer string=w483:string)  [unwired: 1 in]
        n195 = Concatenate Strings(w488, w483) -> (w487:string)
        n196 = Concatenate Strings(w486, w483) -> (w482:string)
        n197 = Concatenate Strings(w485, w483) -> (w481:string)
        n198 = Concatenate Strings(w484, w483) -> (w480:string)
        n199 = call-poly <vilib>:"Write Key.vi"("section"=w476, "value"=w489, "key"=w487, "refnum"=w475) -> ("refnum out"=w474:T1)  [unwired: 2 in, 5 out]
        n200 = call-poly <vilib>:"Write Key.vi"("section"=w476, "value"=w479, "key"=w482, "refnum"=w474) -> ("refnum out"=w473:T1)  [unwired: 2 in, 5 out]
        n201 = call-poly <vilib>:"Write Key.vi"("section"=w476, "value"=w478, "key"=w481, "refnum"=w473) -> ("refnum out"=w472:T1)  [unwired: 1 in, 6 out]
        n202 = call-poly <vilib>:"Write Key.vi"("section"=w476, "value"=w477, "key"=w480, "refnum"=w472) -> ("refnum out"=w471:T1)  [unwired: 1 in, 6 out]
      }
    }
  }
  n203 = call <vilib>:"Close Config Data.vi"("refnum"=w4) -> ("error out"=w5:errorcluster)  [unwired: 2 in, 8 out]
  n204 = call <vilib>:"Simple Error Handler.vi"("error in (no error)"=w5) -> ()  [unwired: 1 in, 8 out]
